vi "RemoveTrailingComma.vi"(2 "Input String":string) -> (7 "Output String":string)   [LabVIEW 2010]
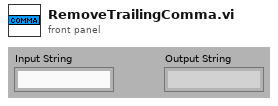
[diagram p1: front panel]
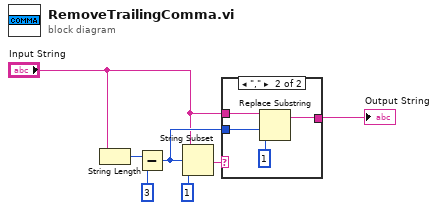
[diagram p0: block diagram]
diagram:
  n1 = String Length(string="Input String") -> (length=w3:i32)
  n2 = Subtract(x=w3, y=3) -> (x-y=w4:i32)
  n3 = String Subset(string="Input String", offset (0)=w4, length (rest)=1 ("length (rest)")) -> (substring=w1:string)
  n4 = case shown="\",\"" w1 {
    tunnel: "Input String" -> [w8 w12]
    tunnel: w4 -> [_ w11]
    tunnel: [w8 w9] -> w7
    frame Default {
    }
    frame "," {
      n5 = Replace Substring(2:1 ("length (len. of substring)"), 3:w11, 5:w12) -> (1:w9:string)  [unwired: 1 in, 1 out]
    }
  }
  "Output String" <- w7
